vi "题目6.4.vi"   [LabVIEW 2017]
uses:
  <vilib>/Utility/file.llb/Write Delimited Spreadsheet (DBL).vi
  <vilib>/measure/NI_MABase.lvlib
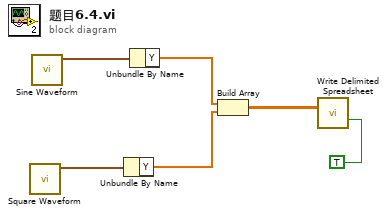
[diagram p0: block diagram]
diagram:
  n1 = call <vilib>:"Square Waveform.vi"() -> ("signal out"=w1:waveform(dbl))  [unwired: 10 in, 1 out]
  n2 = call <vilib>:"Sine Waveform.vi"() -> ("signal out"=w3:waveform(dbl))  [unwired: 10 in, 1 out]
  n3 = Unbundle By Name(w1) -> ("Y"=w6:dbl[])
  n4 = Unbundle By Name(w3) -> ("Y"=w2:dbl[])
  n5 = Build Array(w2, w6) -> (w4:dbl[][])
  n6 = call-poly <vilib>:"Write Delimited Spreadsheet.vi"("2D data"=w4, "append to file? (new file:F)"=TRUE) -> ()  [unwired: 12 in, 2 out]
